vi "Start SubComponent.vi"(5 "Component ID":u8, 7 "FPGA Interface":refnum<class "FPGA Interface.lvclass">, 8 "error in (no error)":errorcluster, 11 "Bus Monitor in":refnum<class "Bus Monitor.lvclass">) -> (0 "error out":errorcluster, 3 "Bus Monitor out":refnum<class "Bus Monitor.lvclass">)   [LabVIEW 2020, in "BCI-1553 API.lvlib" / "Bus Monitor.lvclass"]
uses:
  Bus Monitor.lvclass
  Dependencies/FPGA Interface/FPGA Interface.lvclass
panel:
  out "Master":u16 format="%04x"
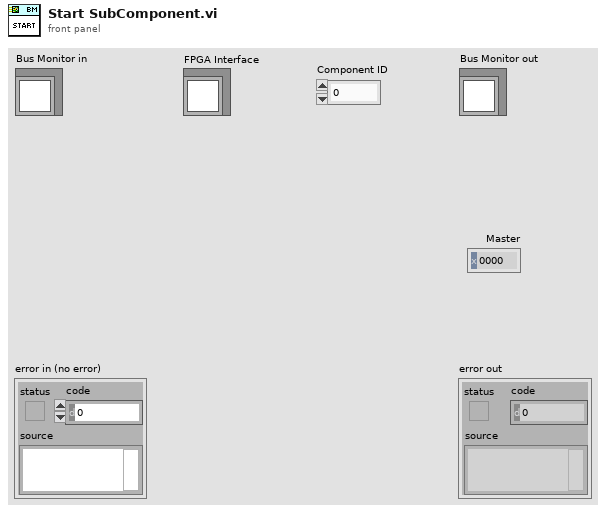
[diagram p1: front panel]
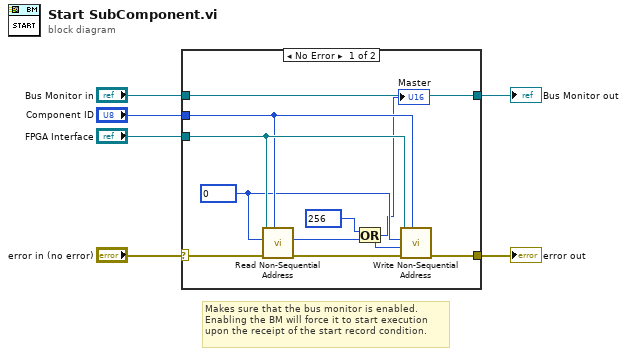
[diagram p0: block diagram]
diagram:
  # "Makes sure that the bus monitor is enabled.\nEnabling the BM will force it to start execution\nupon the receipt of the start record condition."
  n1 = case shown="No Error" "error in (no error)" {
    selector: "error in (no error)" -> [w14 w18]
    tunnel: [w12 w18] -> w1
    tunnel: "Bus Monitor in" -> [w9 w17]
    tunnel: "FPGA Interface" -> [w16 _]
    tunnel: "Component ID" -> [w15 _]
    tunnel: [w9 w17] -> w2
    frame No Error {
      w11 = u16 0 ("Address")
      n2 = call-dynamic "Read Non-Sequential Address.vi"("Target IC (1-8)"=w15, "error in (no error)"=w14, "Address"=w11, "FPGA Interface in"=w16) -> ("error out"=w13:errorcluster, "Data"=w10:u16)  [unwired: 6 in]
      n3 = Or(x=u16 256 ("Address"), y=w10) -> (x .or. y?=w7:u16)
      "Master" <- w7
      n4 = call-dynamic "Write Non-Sequential Address.vi"("Target IC (1-8)"=w15, "error in (no error)"=w13, "Data"=w7, "Address"=w11, "FPGA Interface in"=w16) -> ("error out"=w12:errorcluster)  [unwired: 6 in]
    }
    frame Error {
    }
  }
  "error out" <- w1
  "Bus Monitor out" <- w2
